vi "Remove All.vi"(11 "Collection In":refnum<class "Collection.lvclass">) -> (3 "Collection Out":refnum<class "Collection.lvclass">)   [LabVIEW 2020, in "Collection.lvclass"]
uses:
  Collection.lvclass
  Collection.lvclass/Collection.ctl
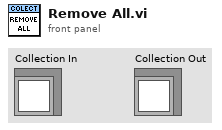
[diagram p1: front panel]
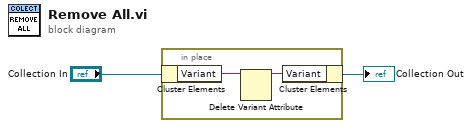
[diagram p0: block diagram]
diagram:
  n1 = in-place {
    n2 = in-place-cluster #1("Collection In") -> ("Variant"=w4:variant)
    n3 = Delete Variant Attribute(7:w4) -> (3:w3:variant)  [unwired: 2 in, 2 out]
    n4 = in-place-cluster #1("Variant"=w3) -> (→"Collection Out":refnum<class "Collection.lvclass">)
  }
